vi "Structure Reporter.vi"() -> ()   [LabVIEW 2023, in "VIDoc Parsing.lvlib" / "Structure Reporter.lvlib"]
uses:
  Structure Reporter.lvlib
  UI Style.vi
  Printers/Confluence Printer/VIDoc Printer - Confluence.lvclass
panel:
  out "Expand String":string
  out "Tree":string(tree)
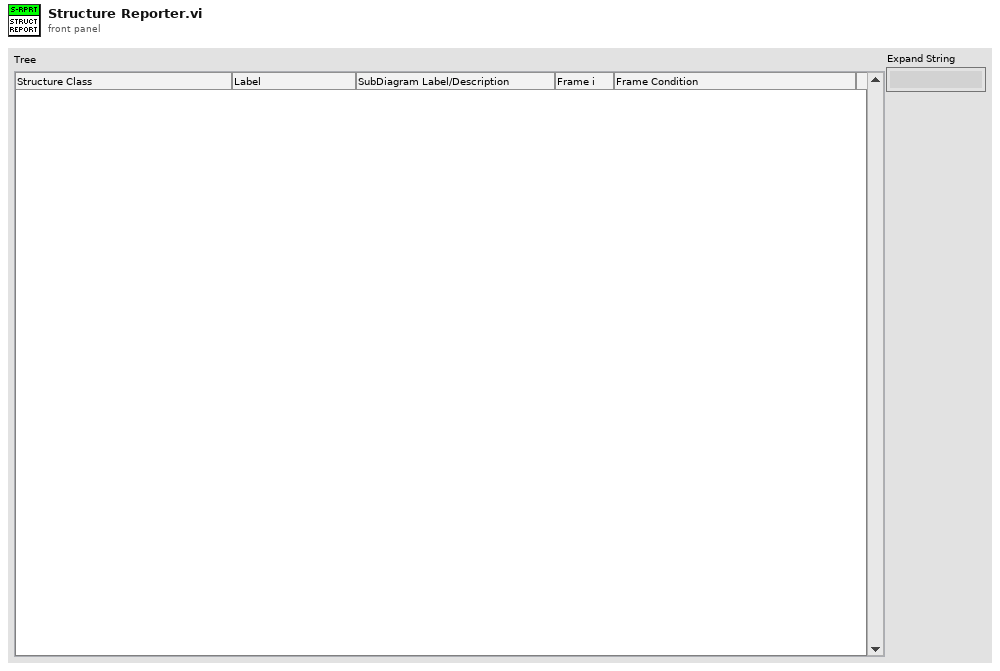
[diagram p1: front panel]
types:
  T1 = typedef "VIDoc Parsing.lvlib/Structure Reporter.lvlib/Structure Result 2.ctl" = cluster{"Depth":i32, "Top":i32, "Left":i32, "Frame index":i32, "Struct":i32, "Object Class Name":string, "Object UID":i32, "Label Visible":bool, "Object Label":string, "SD Label Visible":bool, "Object SD Label":string, "Frame Name":string, "Diag UID":i32, "Owner Class Name":string, "Owner UID":i32, "Diag Struct":i32[], "Parent Struct":i32, "Diag UIDs":i32[], "Tree Name":string, "Diag Ref":refnum<vi>, "Owner Classes":string[], "Owner":refnum<vi>, "Owner UIDs":i32[], "Tag Indent":i32, "Tag Value":i32, "Child Tag":string}
  T2 = typedef "VIDoc Parsing.lvlib/Structure Reporter.lvlib/Tree Cluster.ctl" = cluster{"Object Class Name":string, "Labels":string[], "Child Tag":string, "Item Indent":i32, "Child Only?":bool, "Glyph Index":i32}
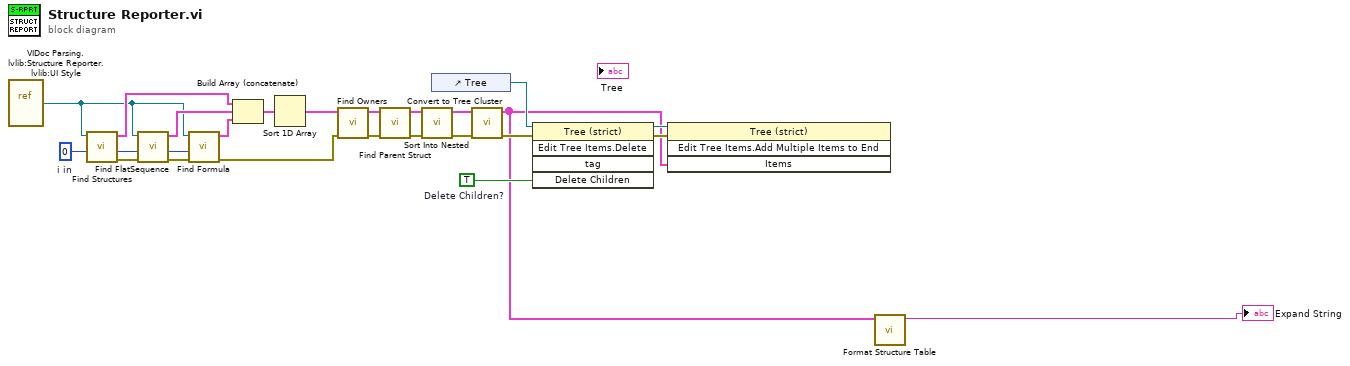
[diagram p0: block diagram]
diagram:
  w6 = TRUE  # Delete Children?
  w24 = 0  # i in
  n1 = vi-ref "VIDoc Parsing.lvlib:Structure Reporter.lvlib:UI Style.vi"() -> (w10:refnum<vi>)
  n2 = call "Find Structures.vi"("i in"=w24, "VI in"=w10) -> ("error out"=w16:errorcluster, "i out"=w23:i32, "Structures"=w25:T1[])  [unwired: 7 in]
  n3 = call "Find FlatSequence.vi"("error in (no error)"=w16, "i in"=w23, "VI in"=w10) -> ("error out"=w15:errorcluster, "i out"=w20:i32, "FlatSequences"=w22:T1[])  [unwired: 6 in]
  n4 = call "Find Formula.vi"("error in (no error)"=w15, "i in"=w20, "VI in"=w10) -> ("error out"=w14:errorcluster, "Array"=w21:T1[])  [unwired: 6 in, 1 out]
  n5 = Build Array (concatenate)(w25, w22, w21) -> (w19:T1[])
  n6 = Sort 1D Array(array=w19) -> (sorted array=w18:T1[])
  n7 = call "Find Owners.vi"("error in (no error)"=w14, "Array in"=w18) -> ("error out"=w13:errorcluster, "Array out"=w17:T1[])  [unwired: 8 in]
  n8 = call "Find Parent Struct.vi"("error in (no error)"=w13, "Objects in"=w17) -> ("error out"=w11:errorcluster, "Found Parent Struct"=w12:T1[])  [unwired: 8 in]
  n9 = call "Sort Into Nested.vi"("error in (no error)"=w11, "Found Parent Struct"=w12) -> ("error out"=w9:errorcluster, "Nested Structures"=w8:T1[])  [unwired: 8 in]
  n10 = control-ref of="Tree"() -> (w4:refnum<vi>)
  n11 = call "Convert to Tree Cluster.vi"("error in (no error)"=w9, "Array in"=w8) -> ("error out"=w5:errorcluster, "Array out"=w2:T2[])  [unwired: 8 in]
  n12 = invoke class="Tree (strict)" method="Edit Tree Items.Delete"(reference=w4, error in=w5, "Delete Children"=w6) -> (reference out=w3:refnum<vi>, error out=w7:errorcluster)  [unwired: 2 in, 3 out]
  n13 = invoke class="Tree (strict)" method="Edit Tree Items.Add Multiple Items to End"(reference=w3, error in=w7, "Items"=w2) -> ()  [unwired: 1 in, 4 out]
  n14 = call "Format Structure Table.vi"("Structure Tree Array in"=w2) -> ("String"=→"Expand String":string)  [unwired: 10 in]
